vi "Verify Parameterized.vi"(5 "Label":string, 7 "Options":refnum<class "Options.lvclass">, 8 "error in":errorcluster, 9 "Set of ctl label -> value var":set{map{string, variant}}(c389), 10 "VI in":refnum<vi>, 11 "TestCase in":refnum<class "TestCase.lvclass">) -> (0 "error out":errorcluster, 3 "TestCase out":refnum<class "TestCase.lvclass">)   [LabVIEW 2026, in "VITester.Extension.lvlib"]
doc: "You pass in a reference to the function you want to test. You also pass in a set of maps. Each map maps each control label to a variant value (You must use the \"to Variant\" primitive or you'll get a broken run arrow due to the type mismatch). The control must be connected to the connector pane. Ideally you would have the same number of elements in your map as controls connected to the connector pane. If you don't specify a value for a control, it just stays whatever the default is set at. The underlying code will cycle through the set and for each map, will set the control values appropriately and then run the vi and capture any indicators connected to the connector pane. The control and corresponding indicator values are all stored in the approved file."
uses:
  VITester.Extension.lvlib
  <vilib>/Addons/_JKI Toolkits/VI Tester/TestCase.llb/TestCase.lvclass
  Approval Tests/Options/Options.lvclass
  Approval Tests/Options/Options.lvclass/Options.ctl
  Approval Tests/Naming Data/Naming Data.lvclass/Naming Data.ctl
  Approval Tests/Naming Data/Read Test VI Name.vi
  Approval Tests/Naming Data/Write Test VI Name.vi
  Approval Tests/Approval Tests.lvlib
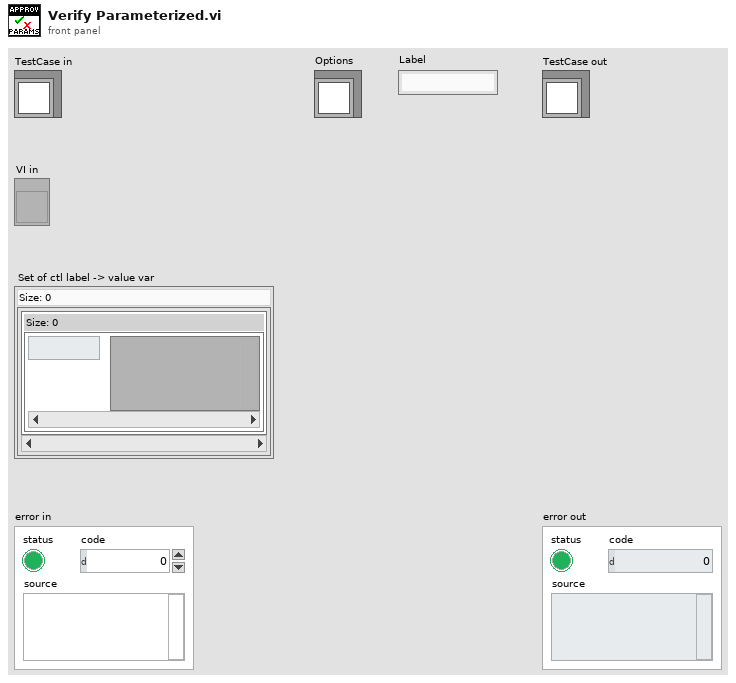
[diagram p1: front panel]
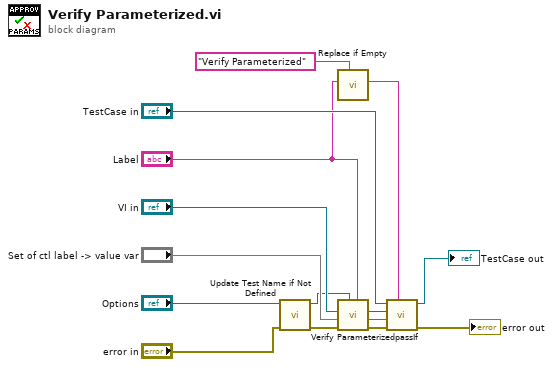
[diagram p0: block diagram]
diagram:
  n1 = call "Update Test Name if Not Defined.vi"("error in"="error in", "Options in"="Options") -> ("error out"=w12:errorcluster, "Options out"=w4:refnum<class "Options.lvclass">)  [unwired: 8 in]
  n2 = call "Replace if Empty.vi"("if empty"="Verify Parameterized", "Text in"="Label") -> ("Text out"=w1:string)  [unwired: 9 in]
  n3 = call "Verify Parameterized.vi"("Label"="Label", "Approval Tests.lvlib:Options.lvclass"=w4, "error in"=w12, "Set of ctl label -> value var"="Set of ctl label -> value var", "VI in"="VI in") -> ("error out"=w14:errorcluster, "Failure Message"=w8:string, "Passed?"=w9:bool)  [unwired: 4 in]
  n4 = call-dynamic "passIf.vi"("custom report message (\"\")"=w1, "error in (no error)"=w14, "message (\"\")"=w8, "pass"=w9, "TestCase in"="TestCase in") -> ("error out"=→"error out":errorcluster, "TestCase out"=→"TestCase out":refnum<class "TestCase.lvclass">)  [unwired: 5 in]
